vi "Process.vi"(8 "error in":errorcluster, 11 "Qbus in":refnum<class "Qbus.lvclass">) -> (0 "error out":errorcluster)   [LabVIEW 2021, in "AudioGenTCPReaderProcess.lvlib"]
uses:
  AudioGenTCPReaderProcess.lvlib
  <vilib>/addons/Qbus/Qbus.lvclass
  <vilib>/NI/STM/TCP/TCP Read Options.ctl
  shared/logger process/controls/event.ctl
  controls/digital generation settings.ctl
  controls/digital protocol settings.ctl
  <vilib>/PDM Acquisition Toolkit/host/Classes/Session/Controls/Logic Levels.ctl
  <vilib>/PDM Acquisition Toolkit/shared/controls/PCM Data Format Configuration.ctl
  <vilib>/PDM Acquisition Toolkit/shared/controls/Digital Edge.ctl
  <vilib>/PDM Acquisition Toolkit/shared/controls/PCM Bit Endianness.ctl
  <vilib>/PDM Acquisition Toolkit/shared/controls/PCM Data Justification.ctl
  <vilib>/PDM Acquisition Toolkit/shared/controls/clock mode.ctl
  <vilib>/PDM Acquisition Toolkit/shared/controls/PCM Frame Sync Control.ctl
  <vilib>/PDM Acquisition Toolkit/host/Classes/Tasks/I2S Output/Control/SignalProperties.ctl
  <vilib>/PDM Acquisition Toolkit/host/Classes/Channels/I2S Ouput/Controls/GenerationChannelProperties.ctl
  <vilib>/NI/STM/TCP/Read Message (TCP).vi
  <vilib>/NI/STM/TCP/Write Message (TCP).vi
  ManageConnection/AudioGenManageConnectionProcess.lvlib
  <vilib>/NI/STM/NI STM.lvlib
  shared/logger process/EventLoggerProcess.lvlib
  Digital Audio Generation/DigitalAudioGenerationProcess.lvlib
  <vilib>/PDM Acquisition Toolkit/host/Classes/Session/DecoderSession.lvclass
  <vilib>/PDM Acquisition Toolkit/shared/PDM Shared.lvlib
  controls/AudioGenTypeDefs.lvlib
  <vilib>/PDM Acquisition Toolkit/host/Classes/Channels/I2S Ouput/I2S Output Channel.lvclass
  <vilib>/PDM Acquisition Toolkit/host/Classes/Tasks/I2S Output/I2S Output Task.lvclass
  subVIs/utility/AudioGenUtility.lvlib
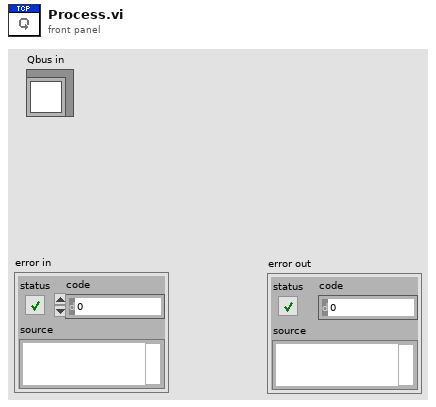
[diagram p1: front panel]
types:
  T1 = typedef "NI STM.lvlib/TCP Read Options.ctl" = cluster{"ignore timeout error":bool, "timeout ms (1000)":i32}
  T2 = typedef "EventLoggerProcess.lvlib/event.ctl" = cluster{"name":string, "description":string}
  T3 = typedef "AudioGenTypeDefs.lvlib/digital generation settings.ctl" = cluster{"data channel list":string, "master clock channel list":string, "digital protocol settings":T4, "signal parameters":T12}
  T4 = typedef "AudioGenTypeDefs.lvlib/digital protocol settings.ctl" = cluster{"logic level":T5, "PCM Data Configuration":T6, "bit clock rate":sgl, "master clock rate":sgl, "clock mode":T10, "Frame Sync Clock Control":T11}
  T5 = typedef "PDM Acquisition Class Library.lvlib/DecoderSession.lvclass/Logic Levels.ctl" = enum16{"3.3 V", "1.8 V", "1.2 V"}
  T6 = typedef "PDM Shared.lvlib/PCM Data Format Configuration.ctl" = cluster{"Frame Sync Edge for Channel 0":T7, "Channel Count Per Frame":u8, "Channel Length":u16, "Bit Depth":u8, "Channel 0 Offset":u16, "Endianness":T8, "Data Justification":T9}
  T7 = typedef "PDM Shared.lvlib/Digital Edge.ctl" = enum8{"Rising", "Falling"}
  T8 = typedef "PDM Shared.lvlib/PCM Bit Endianness.ctl" = enum16{"MSB First", "LSB First"}
  T9 = typedef "PDM Shared.lvlib/PCM Data Justification.ctl" = enum16{"Left Justified", "Right Justified"}
  T10 = typedef "PDM Shared.lvlib/clock mode.ctl" = enum16{"divided clock", "DDS"}
  T11 = typedef "PDM Shared.lvlib/PCM Frame Sync Control.ctl" = cluster{"Frame Length":u16, "Frame Sync Pulse Width":u16, "Bit Clock Edge  Sync":T7}
  T12 = typedef "PDM Acquisition Class Library.lvlib/I2S Output Task.lvclass/SignalProperties.ctl" = cluster{"cyclic signal":dbl[], "channel parameters":T13[]}
  T13 = typedef "PDM Acquisition Class Library.lvlib/I2S Output Channel.lvclass/GenerationChannelProperties.ctl" = cluster{"cyclic period":dbl, "cyclic phase offset":dbl, "gain":dbl}
  T14 = typedef "NI STM.lvlib/TCP Connection Info.ctl" = cluster{"connection ID":refnum<k5>, "meta data":T15[]}
  T15 = typedef "NI STM.lvlib/MetaDataElement.ctl" = string
  T16 = typedef "AudioGenTypeDefs.lvlib/generation status.ctl" = enum16{"idle", "committed", "generating"}
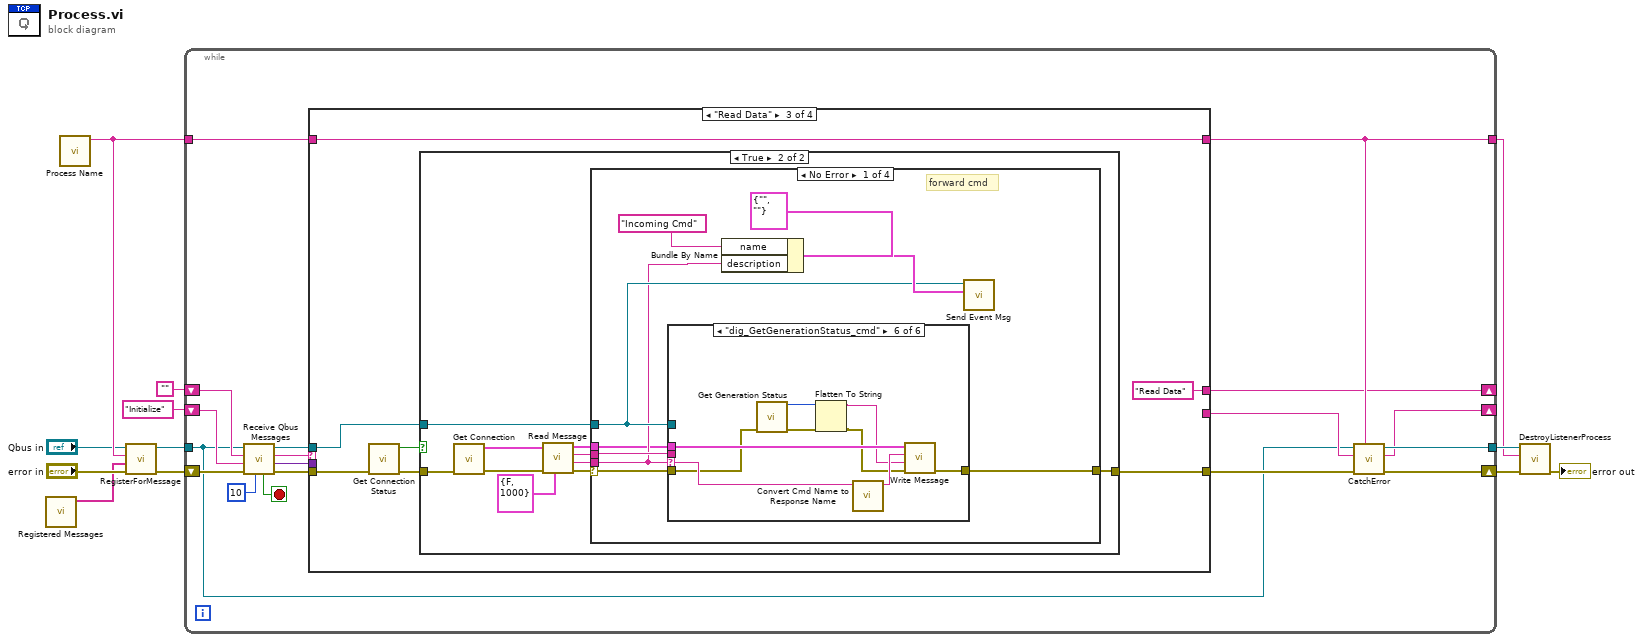
[diagram p0: block diagram]
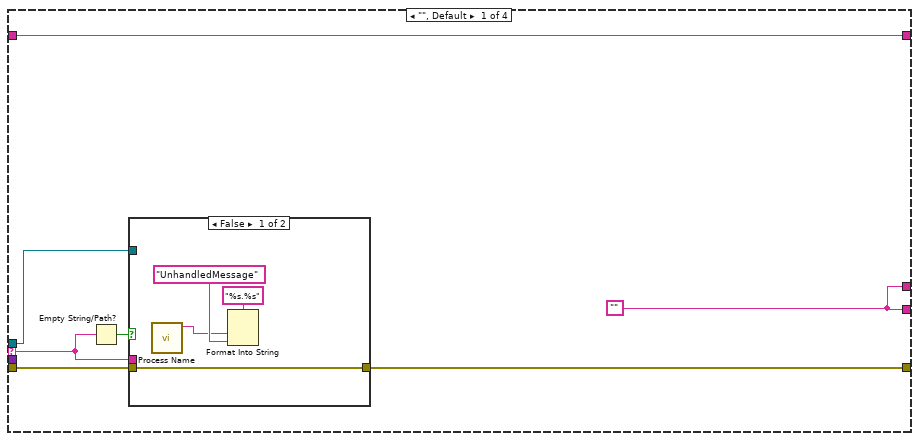
[diagram p2: hidden frame]
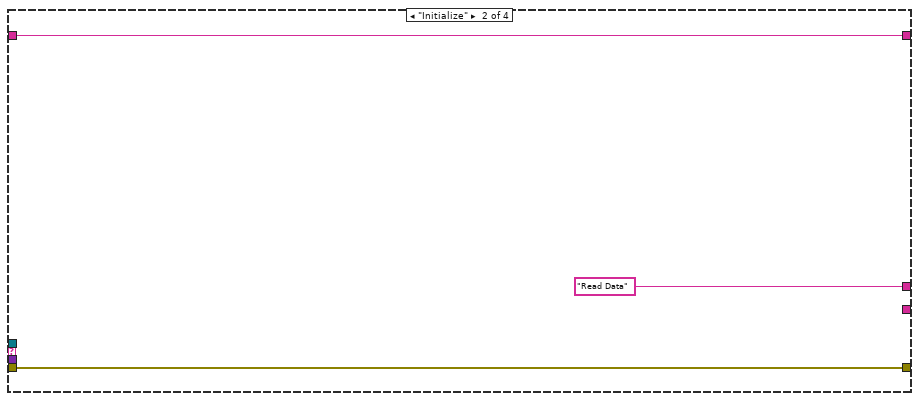
[diagram p4: hidden frame]
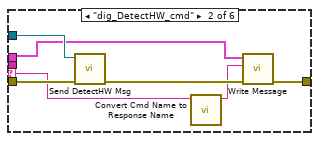
[diagram p7: hidden frame]
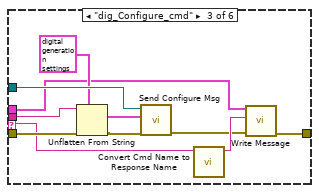
[diagram p8: hidden frame]
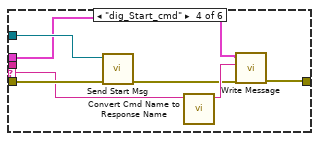
[diagram p9: hidden frame]
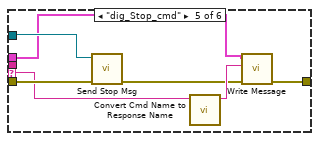
[diagram p10: hidden frame]
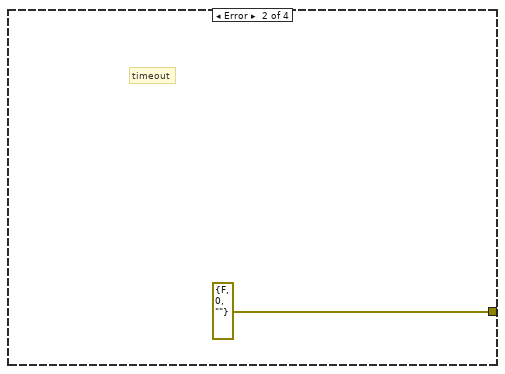
[diagram p11: hidden frame]
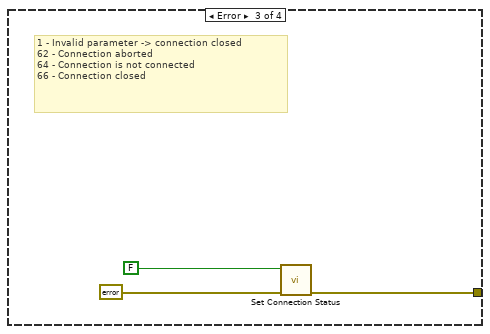
[diagram p12: hidden frame]
diagram:
  n1 = call "Registered Messages.vi"() -> ("registered messages"=w5:string[])  [unwired: 11 in]
  n2 = call "Process Name.vi"() -> ("process name"=w8:string)  [unwired: 11 in]
  n3 = call <vilib>:"RegisterForMessage.vi"("error in (no error)"="error in", "message names"=w5, "process name"=w8, "Qbus in"="Qbus in") -> ("error in (no error)"=w11:errorcluster, "Qbus out"=w12:refnum<class "Qbus.lvclass">)  [unwired: 6 in]
  n4 = while {
    shift-right: [w16] -> _
    shift-left: "" -> [w29]
    tunnel: w12 -> [w14]
    tunnel: w8 -> [w13]
    tunnel: [w23] -> w3
    tunnel: [w18] -> w1
    shift-right: [w22] -> _
    shift-left: "Initialize" -> [w25]
    shift-right: [w24] -> w4
    shift-left: w11 -> [w21]
    stop <- w30 stop-if-true
    n5 = call "Receive Qbus Messages.vi"("timeout(ms)"=10 ("milliseconds to wait"), "error in (no error)"=w21, "priority action"=w25, "default action"=w29, "Qbus in"=w14) -> ("error out"=w28:errorcluster, "message value"=w26:variant, "action"=w20:string, "Qbus out"=w27:refnum<class "Qbus.lvclass">, "exit"=w30:bool)  [unwired: 2 in]
    n6 = case shown="\"Read Data\"" w20 {
      selector: w20 -> [w34 _ _ _]
      tunnel: w28 -> [w36 w45 w51 w121]
      tunnel: w27 -> [w32 _ w47 _]
      tunnel: [w35 w45 w46 w121] -> w15
      tunnel: w26 -> [_ _ _ _]
      tunnel: [w37 w44 w52 w120] -> w18
      tunnel: w13 -> [w37 w44 w52 w120]
      tunnel: [w31 _ _ _] -> w17
      tunnel: [w31 "Read Data" "Read Data" _] -> w16
      frame "", Default {
        w31 = ""
        n7 = Empty String/Path?(string/path=w34) -> (empty?=w33:bool)
        n8 = case shown="False" w33 {
          tunnel: [w38 w42] -> w35
          tunnel: w36 -> [w38 w42]
          tunnel: w34 -> [_ _]
          tunnel: w32 -> [_ _]
          frame False {
            n9 = call "Process Name.vi"() -> ("process name"=w39:string)  [unwired: 11 in]
            n10 = Format Into String(format string="%s.%s", w39, "UnhandledMessage" ("ProcessName")) -> ()  [unwired: 2 in, 2 out]
          }
          frame True {
          }
        }
      }
      frame "Initialize" {
      }
      frame "Read Data" {
        n11 = call "Get Connection Status.vi"("error in (no error)"=w51) -> ("error out"=w49:errorcluster, "connected"=w50:bool)  [unwired: 9 in]
        n12 = case shown="True" w50 {
          tunnel: w49 -> [w53 w63]
          tunnel: [w53 w57] -> w46
          tunnel: w47 -> [_ w60]
          frame False {
          }
          frame True {
            n13 = call "Get Connection.vi"("error in (no error)"=w63) -> ("error out"=w62:errorcluster, "connection"=w61:T14)  [unwired: 9 in]
            n14 = call-poly <vilib>:"Read Message.vi"("options"=T1 {"ignore timeout error"=FALSE, "timeout ms (1000)"=1000}, "error in"=w62, "connection info in"=w61) -> ("error out"=w55:errorcluster, "name"=w58:T15, "data string"=w59:string, "connection info out"=w54:T14)  [unwired: 3 in, 2 out]
            n15 = case shown="No Error" w55 {
              selector: w55 -> [w68 _ _ w119]
              tunnel: w60 -> [w69 _ _ _]
              tunnel: w59 -> [w67 _ _ _]
              tunnel: w58 -> [w66 _ _ _]
              tunnel: [w64 errorcluster {"status"=FALSE, "code"=0, "source"=""} ("error out") w118 w119] -> w57
              tunnel: w54 -> [w65 _ _ _]
              frame No Error {
                # "forward cmd"
                n16 = case shown="\"dig_GetGenerationStatus_cmd\"" w66 {
                  selector: w66 -> [_ w75 w82 w92 w99 w111]
                  tunnel: w68 -> [w73 w80 w90 w98 w104 w110]
                  tunnel: [w73 w77 w81 w94 w101 w112] -> w64
                  tunnel: w69 -> [_ w79 w91 w97 w105 _]
                  tunnel: w67 -> [_ _ w88 _ _ _]
                  tunnel: w65 -> [_ w76 w83 w93 w100 w113]
                  frame "", Default {
                  }
                  frame "dig_DetectHW_cmd" {
                    n17 = call "Send DetectHW Msg.vi"("error in"=w80, "Qbus in"=w79) -> ("error out"=w78:errorcluster)  [unwired: 8 in, 1 out]
                    n18 = call "Convert Cmd Name to Response Name.vi"("cmd name"=w75) -> ("response name"=w74:string)  [unwired: 10 in]
                    n19 = call-poly <vilib>:"Write Message.vi"("error in"=w78, "name"=w74, "connection info in"=w76) -> ("error out"=w77:errorcluster)  [unwired: 7 in, 1 out]
                  }
                  frame "dig_Configure_cmd" {
                    n20 = Unflatten From String(type=T3 {"data channel list"="", "master clock channel list"="", "digital protocol settings"={"logic level"=enum."3.3 V", "PCM Data Configuration"={"Frame Sync Edge for Channel 0"=enum."Falling", "Channel Count Per Frame"=2, "Channel Length"=32, "Bit Depth"=24, "Channel 0 Offset"=1, "Endianness"=enum."MSB First", "Data Justification"=enum."Left Justified"}, "bit clock rate"=3025000.0, "master clock rate"=3025000.0, "clock mode"=enum."divided clock", "Frame Sync Clock Control"={"Frame Length"=64, "Frame Sync Pulse Width"=32, "Bit Clock Edge  Sync"=enum."Falling"}}, "signal parameters"={"cyclic signal"=[], "channel parameters"=[]}} ("digital generation"), binary string=w88, error in (no error)=w90) -> (value=w86:T3, error out=w89:errorcluster)  [unwired: 2 in, 1 out]
                    n21 = call "Send Configure Msg.vi"("error in"=w89, "digital generation"=w86, "Qbus in"=w91) -> ("error out"=w84:errorcluster)  [unwired: 7 in, 1 out]
                    n22 = call "Convert Cmd Name to Response Name.vi"("cmd name"=w82) -> ("response name"=w85:string)  [unwired: 10 in]
                    n23 = call-poly <vilib>:"Write Message.vi"("error in"=w84, "name"=w85, "connection info in"=w83) -> ("error out"=w81:errorcluster)  [unwired: 7 in, 1 out]
                  }
                  frame "dig_Start_cmd" {
                    n24 = call "Send Start Msg.vi"("error in"=w98, "Qbus in"=w97) -> ("error out"=w95:errorcluster)  [unwired: 8 in, 1 out]
                    n25 = call "Convert Cmd Name to Response Name.vi"("cmd name"=w92) -> ("response name"=w96:string)  [unwired: 10 in]
                    n26 = call-poly <vilib>:"Write Message.vi"("error in"=w95, "name"=w96, "connection info in"=w93) -> ("error out"=w94:errorcluster)  [unwired: 7 in, 1 out]
                  }
                  frame "dig_Stop_cmd" {
                    n27 = call "Send Stop Msg.vi"("error in"=w104, "Qbus in"=w105) -> ("error out"=w102:errorcluster)  [unwired: 8 in, 1 out]
                    n28 = call "Convert Cmd Name to Response Name.vi"("cmd name"=w99) -> ("response name"=w103:string)  [unwired: 10 in]
                    n29 = call-poly <vilib>:"Write Message.vi"("error in"=w102, "name"=w103, "connection info in"=w100) -> ("error out"=w101:errorcluster)  [unwired: 7 in, 1 out]
                  }
                  frame "dig_GetGenerationStatus_cmd" {
                    n30 = call "Get Generation Status.vi"("error in (no error)"=w110) -> ("error out"=w109:errorcluster, "generation status"=w108:T16)  [unwired: 9 in]
                    n31 = Flatten To String(anything=w108, error in (no error)=w109) -> (data string=w107:string, error out=w106:errorcluster)  [unwired: 2 in, 1 out]
                    n32 = call "Convert Cmd Name to Response Name.vi"("cmd name"=w111) -> ("response name"=w114:string)  [unwired: 10 in]
                    n33 = call-poly <vilib>:"Write Message.vi"("error in"=w106, "data"=w107, "name"=w114, "connection info in"=w113) -> ("error out"=w112:errorcluster)  [unwired: 6 in, 1 out]
                  }
                }
                n34 = Bundle By Name(cluster=T2 {"name"="", "description"=""} ("event"), "name"="Incoming Cmd", "description"=w66) -> (w70:T2)
                n35 = call "Send Event Msg.vi"("event"=w70, "Qbus in"=w69) -> ()  [unwired: 8 in, 2 out]
              }
              frame Error {
                # "timeout"
              }
              frame Error {
                # "1 - Invalid parameter -> connection closed\n62 - Connection aborted\n64 - Connection is not connected\n66 - Connection closed"
                n36 = call "Set Connection Status.vi"("error in (no error)"=errorcluster {"status"=FALSE, "code"=0, "source"=""}, "connected"=FALSE) -> ("error out"=w118:errorcluster)  [unwired: 9 in]
              }
              frame Default {
              }
            }
          }
        }
      }
      frame "Exit" {
      }
    }
    n37 = call <vilib>:"CatchError.vi"("source"=w18, "error in (no error)"=w15, "next action in"=w17, "Qbus in"=w14) -> ("error out"=w24:errorcluster, "next action out"=w22:string, "Qbus out"=w23:refnum<class "Qbus.lvclass">)  [unwired: 5 in]
  }
  n38 = call <vilib>:"DestroyListenerProcess.vi"("error in (no error)"=w4, "process name"=w1, "Qbus in"=w3) -> ("error in (no error)"=→"error out":errorcluster)  [unwired: 7 in, 1 out]
